vi "Untitled 1.vi"() -> ()   [LabVIEW 2017]
uses:
  <vilib>/addons/internet/NI_InternetTK_Core_VIs.lvlib
panel:
  out "full document URL":string
  out "content":string
  in  "string":string="/current"
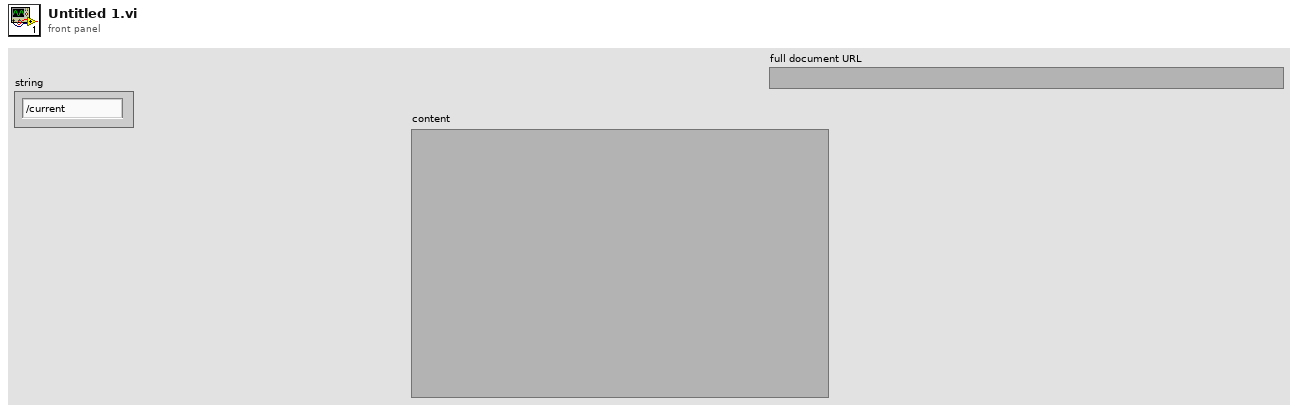
[diagram p1: front panel]
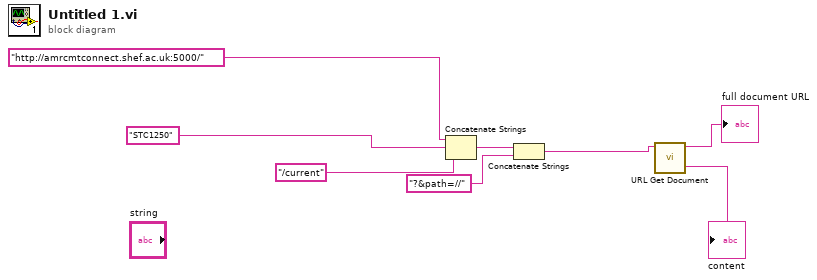
[diagram p0: block diagram]
diagram:
  n1 = Concatenate Strings("http://amrcmtconnect.shef.ac.uk:5000/" ("MT Connect Agent 2"), "STC1250" ("Machine 2"), "/current" ("string")) -> (w8:string)
  n2 = Concatenate Strings(w8, "?&path=//" ("string")) -> (w3:string)
  n3 = call <vilib>:"URL Get Document.vi"("URL"=w3) -> ("full document URL"=→"full document URL":string, "content"=→"content":string)  [unwired: 6 in, 3 out]
